vi "Kinimatics_Calculate Trig for dTheta.vi"(11 "DTHETA":dbl) -> (0 "Cos Of DTheta Out":dbl, 1 "Sin Of DTheta Out":dbl, 2 "Cosine/dTheta Out":dbl, 3 "Sin/dTheta Out":dbl)   [LabVIEW 2020, in "Swerve_Odometry_SEN.lvlib"]
uses:
  Swerve_Odometry_SEN.lvlib
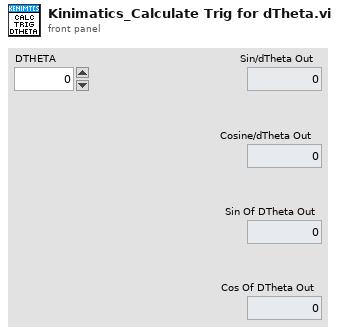
[diagram p1: front panel]
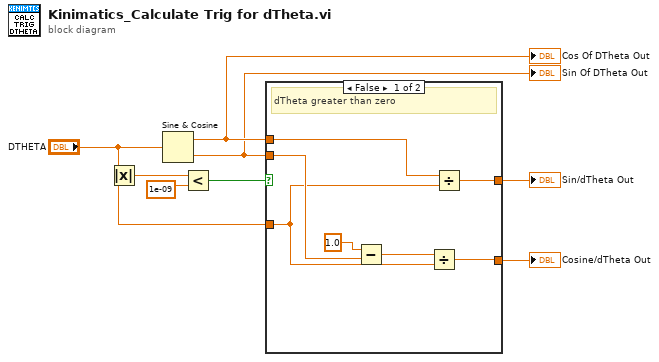
[diagram p0: block diagram]
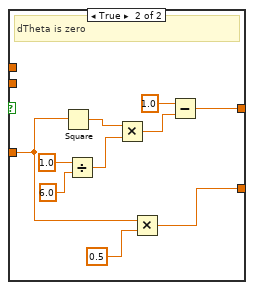
[diagram p2: hidden frame]
diagram:
  n1 = Absolute Value(x="DTHETA") -> (abs(x)=w2:dbl)
  n2 = Sine & Cosine(0:"DTHETA") -> (1:w8:dbl, 2:w6:dbl)
  "Cos Of DTheta Out" <- w8
  "Sin Of DTheta Out" <- w6
  n3 = Less?(x=w2, y=1e-09) -> (x < y?=w3:bool)
  n4 = case shown="False" w3 {
    tunnel: "DTHETA" -> [w9 w17]
    tunnel: [w14 w19] -> w5
    tunnel: [w11 w16] -> w4
    tunnel: w8 -> [w15 _]
    tunnel: w6 -> [w12 _]
    frame False {
      # "dTheta greater than zero"
      n5 = Subtract(x=1.0, y=w12) -> (x-y=w10:dbl)
      n6 = Divide(x=w10, y=w9) -> (x/y=w11:dbl)
      n7 = Divide(x=w15, y=w9) -> (x/y=w14:dbl)
    }
    frame True {
      # "dTheta is zero"
      n8 = Square(x=w17) -> (x^2=w22:dbl)
      n9 = Divide(x=1.0, y=6.0) -> (x/y=w21:dbl)
      n10 = Multiply(x=w22, y=w21) -> (x*y=w20:dbl)
      n11 = Multiply(x=w17, y=0.5) -> (x*y=w16:dbl)
      n12 = Subtract(x=1.0, y=w20) -> (x-y=w19:dbl)
    }
  }
  "Sin/dTheta Out" <- w5
  "Cosine/dTheta Out" <- w4
